vi "Read I2C.vi"(8 "error in (no error)":errorcluster, 11 "LPS25H(B) in":refnum<class "LPS25H(B).lvclass">) -> (0 "error out":errorcluster, 2 "LINX I2C":refnum<class "LINX I2C.lvclass">, 3 "LPS25H(B) out":refnum<class "LPS25H(B).lvclass">)   [LabVIEW 2020, in "LPS25H(B).lvclass"]
uses:
  LPS25H(B).lvclass
  LINX I2C/LINX I2C.lvclass
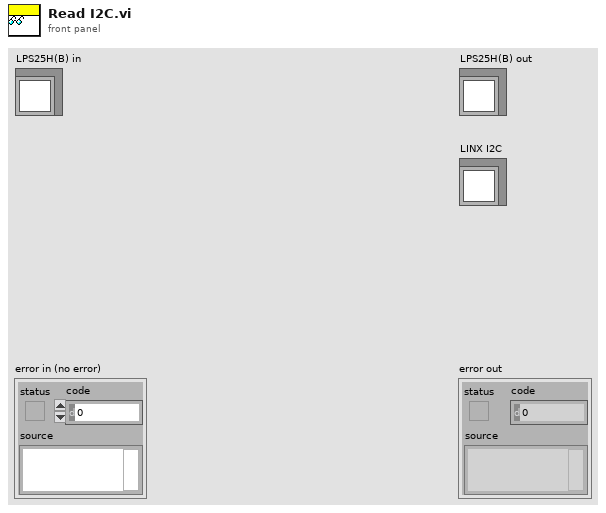
[diagram p1: front panel]
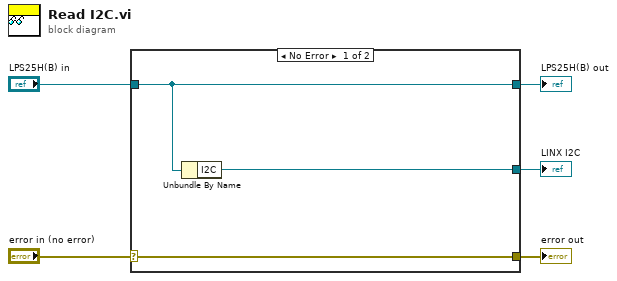
[diagram p0: block diagram]
diagram:
  n1 = case shown="No Error" "error in (no error)" {
    selector: "error in (no error)" -> [w8 w9]
    tunnel: [w8 w9] -> w4
    tunnel: [w7 w10] -> w2
    tunnel: "LPS25H(B) in" -> [w7 w10]
    tunnel: [w6 _] -> w1
    frame No Error {
      n2 = Unbundle By Name(w7) -> ("I2C"=w6:refnum<class "LINX I2C.lvclass">)
    }
    frame Error {
    }
  }
  "error out" <- w4
  "LPS25H(B) out" <- w2
  "LINX I2C" <- w1
